vi "populateEventDetailedState.vi"(8 "error in (no error)":errorcluster, 11 "Model in":refnum<class "Model.lvclass">) -> (0 "error out":errorcluster, 3 "Model out":refnum<class "Model.lvclass">)   [LabVIEW 2016, in "Model.lvclass"]
uses:
  Model.lvclass
  Model.lvclass/Model.ctl
  Publisher/Publisher.lvclass/Publisher.ctl
  Publisher/Publisher.lvclass
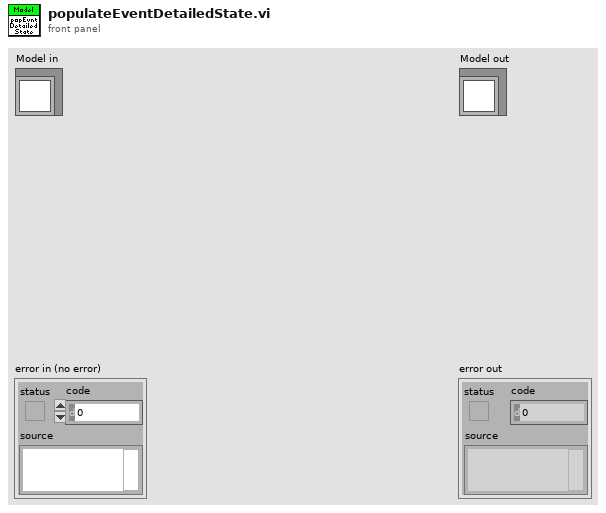
[diagram p1: front panel]
types:
  T1 = typedef "M1M3SupportTopics.lvlib/DetailedStates.ctl" = enum16{"OfflineState", "InitialState", "StandbyState", "DisabledState", "ParkedState", "FaultState", "ParkedMaintenanceState", "ActiveMaintenanceState"}
  T2 = typedef "M1M3SupportTopics.lvlib/Timestamp.ctl" = dbl
  T3 = typedef "M1M3SupportTopics.lvlib/EventDetailedState.ctl" = cluster{"Timestamp":T2, "DetailedStates":T1}
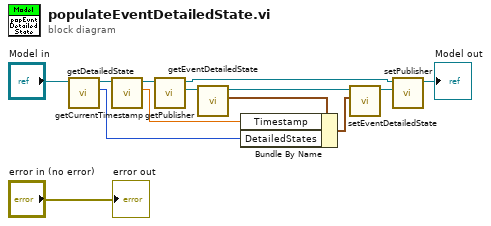
[diagram p0: block diagram]
diagram:
  n1 = call "getDetailedState.vi"("Model in"="Model in") -> ("DetailedStates"=w1:T1, "Model out"=w2:refnum<class "Model.lvclass">)  [unwired: 9 in]
  n2 = call "getCurrentTimestamp.vi"("Model in"=w2) -> ("Timestamp"=w12:T2, "Model out"=w13:refnum<class "Model.lvclass">)  [unwired: 8 in, 1 out]
  n3 = call "getPublisher.vi"("Model in"=w13) -> ("Publisher"=w8:refnum<class "Publisher.lvclass">, "Model out"=w11:refnum<class "Model.lvclass">)  [unwired: 9 in]
  n4 = call "getEventDetailedState.vi"("Publisher in"=w8) -> ("EventDetailedState"=w7:T3, "Publisher out"=w6:refnum<class "Publisher.lvclass">)  [unwired: 9 in]
  n5 = Bundle By Name(cluster=w7, "Timestamp"=w12, "DetailedStates"=w1) -> (w5:T3)
  n6 = call "setEventDetailedState.vi"("EventDetailedState"=w5, "Publisher in"=w6) -> ("Publisher out"=w4:refnum<class "Publisher.lvclass">)  [unwired: 9 in]
  n7 = call "setPublisher.vi"("Publisher"=w4, "Model in"=w11) -> ("Model out"=→"Model out":refnum<class "Model.lvclass">)  [unwired: 9 in]
  "error out" <- "error in (no error)"
